vi "reagent volumes.vi"(9 "Index Values":u32[](array[numeric]), 10 "State Settings":T4[][](array[typedef]) {"valve cycle time" min=0.2 step=0.1 format="%.2f"; "flow division"."5" min=0.0 max=1.0 step=0.01 format="%.3f"; "flow division"."4" min=0.0 max=1.0 step=0.01 format="%.3f"; "flow division"."3" min=0.0 max=1.0 step=0.01 format="%.3f"; "flow division"."2" min=0.0 max=1.0 step=0.01 format="%.3f"; "flow division"."1" min=0.0 max=1.0 step=0.01 format="%.3f"; "flow rate" format="%.3f"}, 11 "Which volumes":T1(ring)) -> (2 "total run time":dbl[unit] format="%<%H:%M:%S%0u>t", 3 "tanks":T2 {"Tank 5" scale format="%.1f"; "Tank 4" scale format="%.1f"; "Tank 3" scale format="%.1f"; "Tank 2" scale format="%.1f"; "Tank 1" scale format="%.1f"})   [LabVIEW 2012]
uses:
  State Setting.ctl
  Stamp/Switch settings vertical.ctl
  flow fraction.ctl
  tanks.ctl
  tank.ctl
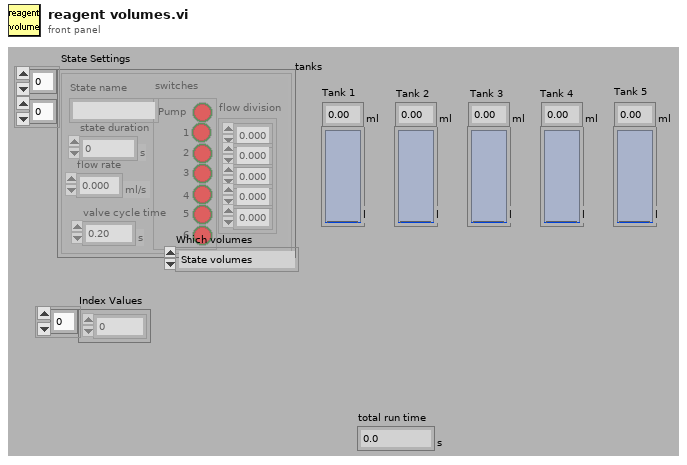
[diagram p1: front panel]
types:
  T1 = enum16{"State volumes", "Cycle volumes", "Experiment volumes"}
  T2 = typedef "tanks.ctl" = cluster{"Tank 1":T3, "Tank 2":T3, "Tank 3":T3, "Tank 4":T3, "Tank 5":T3}
  T3 = typedef "tank.ctl" = dbl[unit]
  T4 = typedef "State Setting.ctl" = cluster{"switches":T5, "flow rate":dbl[unit], "flow division":cluster{"1":T6, "2":T6, "3":T6, "4":T6, "5":T6}, "State name":string, "state duration":dbl[unit], "valve cycle time":dbl[unit]}
  T5 = typedef "Switch settings vertical.ctl" = cluster{"Pump":bool, "1":bool, "2":bool, "3":bool, "4":bool, "5":bool, "6":bool}
  T6 = typedef "flow fraction.ctl" = dbl
  T7 = cluster{"1":dbl[unit], "2":dbl[unit], "3":dbl[unit], "4":dbl[unit], "5":dbl[unit]}
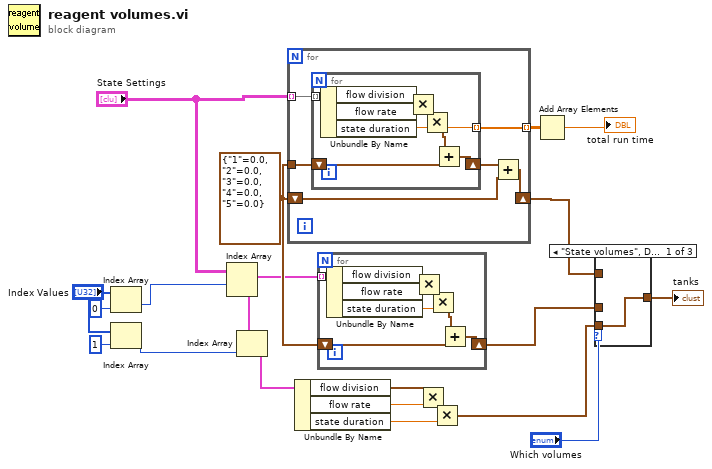
[diagram p0: block diagram]
diagram:
  w12 = T7 {"1"=0.0, "2"=0.0, "3"=0.0, "4"=0.0, "5"=0.0}
  n1 = Index Array(array="Index Values", index=0) -> (element=w6:u32)
  n2 = Index Array(array="Index Values", index=1) -> (element=w4:u32)
  n3 = Index Array(array="State Settings", index (row)=w6) -> (element=w5:T4[])  [unwired: 1 in]
  n4 = Index Array(array=w5, index=w4) -> (element=w3:T4)
  n5 = for {
    tunnel: "State Settings" -> [w26] mode=indexing
    shift-right: [w24] -> w9
    shift-left: w12 -> [w23]
    tunnel: w12 -> [w22]
    tunnel: [w21] -> w11 mode=indexing
    n6 = for {
      tunnel: w26 -> [w34] mode=indexing
      shift-right: [w28] -> w25
      shift-left: w22 -> [w27]
      tunnel: [w31] -> w21 mode=indexing
      n7 = Unbundle By Name(w34) -> ("flow division"=w29:cluster{"1":T6, "2":T6, "3":T6, "4":T6, "5":T6}, "flow rate"=w33:dbl[unit], "state duration"=w31:dbl[unit])
      n8 = Multiply(x=w29, y=w33) -> (x*y=w32:T7)
      n9 = Multiply(x=w32, y=w31) -> (x*y=w30:T7)
      n10 = Add(x=w30, y=w27) -> (x+y=w28:T7)
    }
    n11 = Add(x=w25, y=w23) -> (x+y=w24:T7)
  }
  n12 = Unbundle By Name(w3) -> ("flow division"=w16:cluster{"1":T6, "2":T6, "3":T6, "4":T6, "5":T6}, "flow rate"=w13:dbl[unit], "state duration"=w15:dbl[unit])
  n13 = for {
    tunnel: w5 -> [w42] mode=indexing
    shift-right: [w36] -> w2
    shift-left: w12 -> [w35]
    n14 = Unbundle By Name(w42) -> ("flow division"=w37:cluster{"1":T6, "2":T6, "3":T6, "4":T6, "5":T6}, "flow rate"=w41:dbl[unit], "state duration"=w39:dbl[unit])
    n15 = Multiply(x=w37, y=w41) -> (x*y=w40:T7)
    n16 = Multiply(x=w40, y=w39) -> (x*y=w38:T7)
    n17 = Add(x=w38, y=w35) -> (x+y=w36:T7)
  }
  n18 = Multiply(x=w16, y=w13) -> (x*y=w14:T7)
  n19 = Multiply(x=w14, y=w15) -> (x*y=w8:T7)
  n20 = Add Array Elements(numeric array=w11) -> (sum=→"total run time":dbl[unit])
  n21 = case shown="\"State volumes\", Default" "Which volumes" {
    tunnel: w9 -> [_ _ w45]
    tunnel: w8 -> [w43 _ _]
    tunnel: w2 -> [_ w44 _]
    tunnel: [w43 w44 w45] -> w1
    frame "State volumes", Default {
    }
    frame "Cycle volumes" {
    }
    frame "Experiment volumes" {
    }
  }
  "tanks" <- w1
